vi "get root path.vi"(8 "error in (no error)":errorcluster, 11 "CCS_Log File in":refnum<class "CCS_Log File.lvclass">) -> (0 "error out":errorcluster, 2 "machine path":path, 3 "CCS_Log File out":refnum<class "CCS_Log File.lvclass">)   [LabVIEW 2018, in "CCS_Log File.lvclass"]
uses:
  CCS_Log File.lvclass
  <vilib>/Utility/config.llb/Read Key (String).vi
  <vilib>/Utility/config.llb/Read Key (U32).vi
  <vilib>/Utility/config.llb/NI_LVConfig.lvlib
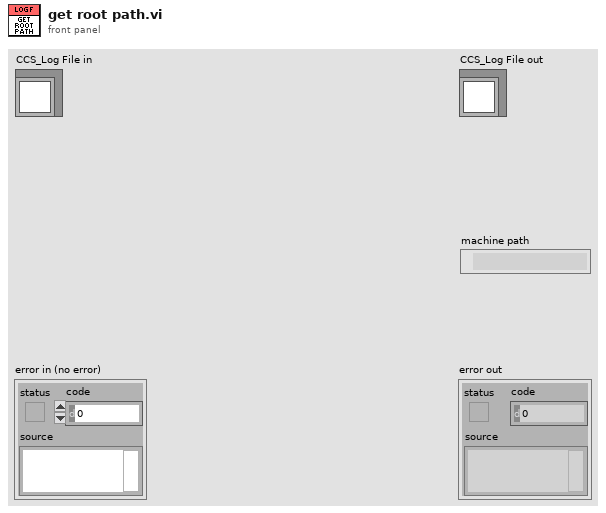
[diagram p1: front panel]
types:
  T1 = typedef "NI_LVConfig.lvlib/Config Data RefNum.ctl" = refnum<k1>
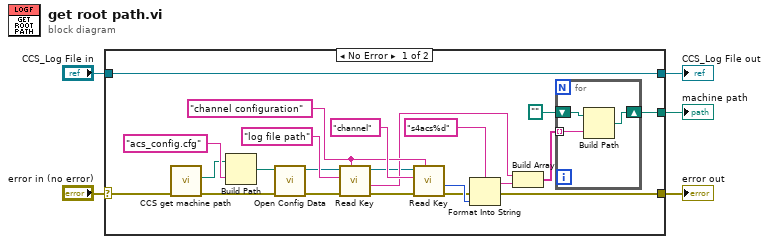
[diagram p0: block diagram]
diagram:
  n1 = case shown="No Error" "error in (no error)" {
    selector: "error in (no error)" -> [w22 w32]
    tunnel: [w11 w32] -> w4
    tunnel: [w27 w31] -> w2
    tunnel: "CCS_Log File in" -> [w27 w31]
    tunnel: [w9 _] -> w1
    frame No Error {
      w19 = "channel configuration"
      n2 = call "CCS get machine path.vi"("error in (no error) 2"=w22) -> ("error in (no error)"=w24:errorcluster, "machine path"=w23:path)  [unwired: 9 in]
      n3 = Build Path(base path=w23, name or relative path="acs_config.cfg") -> (appended path=w26:path)
      n4 = call <vilib>:"Open Config Data.vi"("error in (no error)"=w24, "configuration file path"=w26) -> ("error out"=w18:errorcluster, "refnum"=w7:T1)  [unwired: 7 in, 1 out]
      n5 = call-poly <vilib>:"Read Key.vi"("section"=w19, "error in (no error)"=w18, "key"="log file path", "refnum"=w7) -> ("error out"=w17:errorcluster, "value"=w16:string, "refnum out"=w6:T1)  [unwired: 4 in, 1 out]
      n6 = call-poly <vilib>:"Read Key.vi"("section"=w19, "error in (no error)"=w17, "key"="channel", "refnum"=w6) -> ("error out"=w12:errorcluster, "value"=w14:u32)  [unwired: 4 in, 2 out]
      n7 = Format Into String(format string="s4acs%d", error in=w12, w14) -> (resulting string=w13:string, error out=w11:errorcluster)  [unwired: 1 in]
      n8 = Build Array(w16, w13) -> (w8:string[])
      n9 = for {
        shift-right: [w30] -> w9
        shift-left: path "" -> [w29]
        tunnel: w8 -> [w28] mode=indexing
        n10 = Build Path(base path=w29, name or relative path=w28) -> (appended path=w30:path)
      }
    }
    frame Error {
    }
  }
  "error out" <- w4
  "CCS_Log File out" <- w2
  "machine path" <- w1
